vi "Device cluster to publisher cluster.vi"(8 "error in":errorcluster, 9 "Device cluster from subVi/Dll":T3, 11 "old Data cluster":T1) -> (0 "errorout":errorcluster, 3 "Data cluster out":T1)   [LabVIEW 2013]
uses:
  dataCluster.ctl
  <vilib>/vision/Image Controls.llb/IMAQ Image.ctl
  DataQueueTypeDef.ctl
  PolyRead/StringRead.vi
  PolyRead/ErrorRead.vi
  PolyRead/u32Read.vi
  PolyRead/PathRead.vi
  PolyRead/I32Read.vi
  PolyRead/BooleanRead.vi
  PolyRead/I32refRead.vi
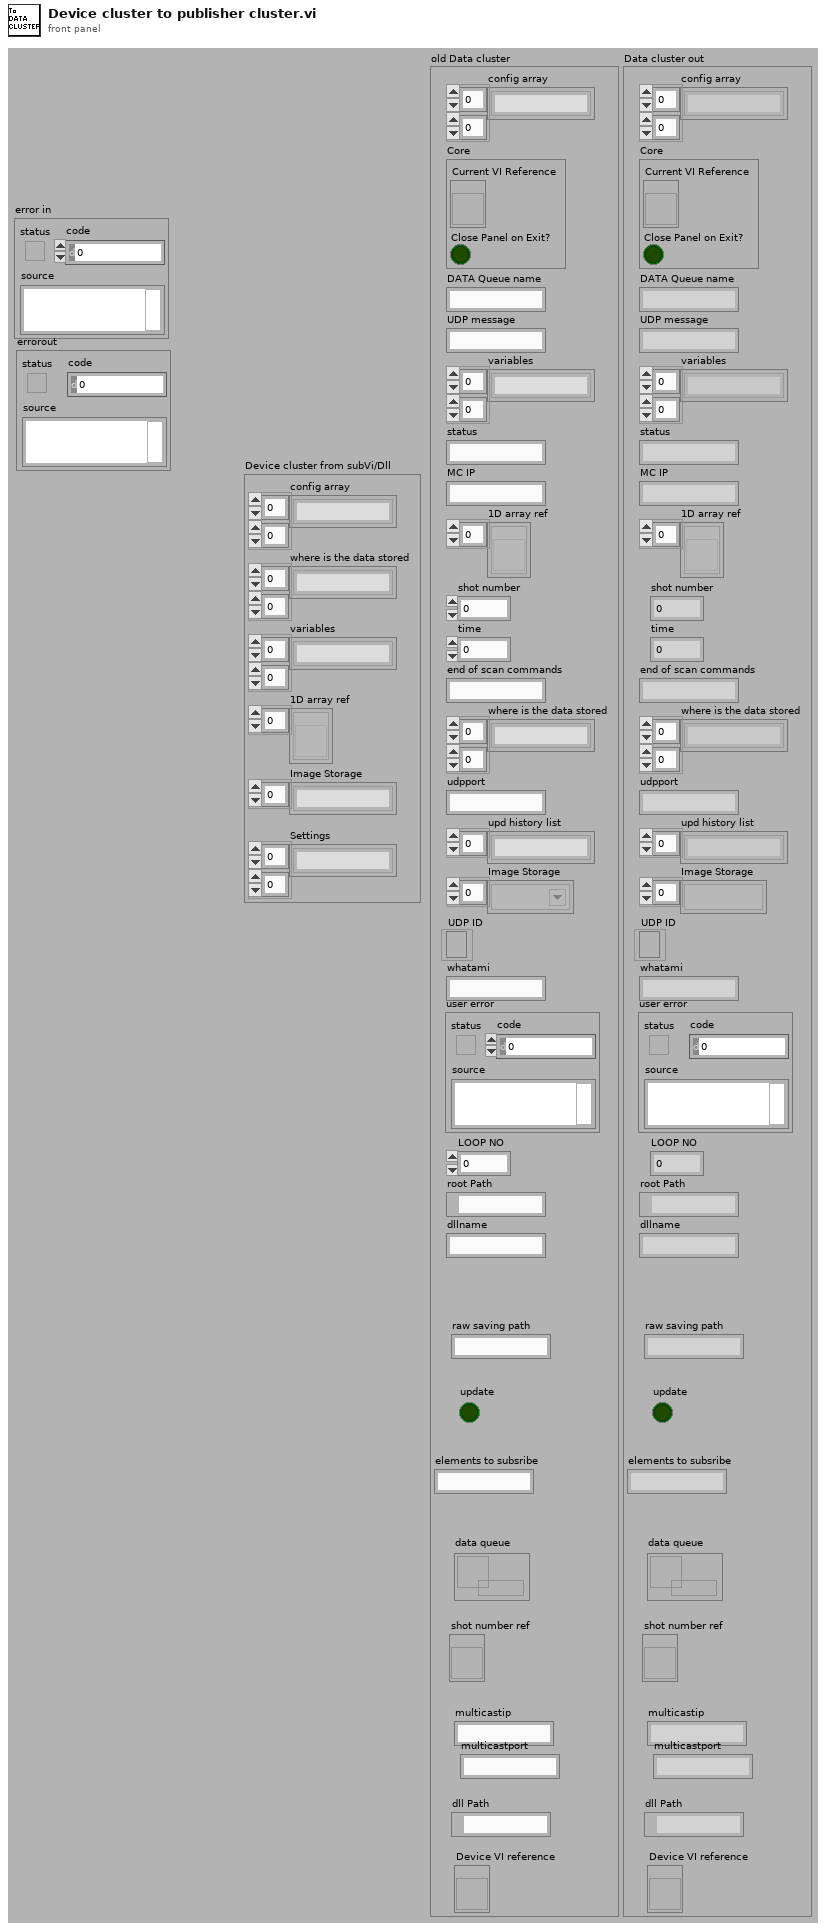
[diagram p1: front panel]
types:
  T1 = typedef "dataCluster.ctl" = cluster{"config array":string[][], "Core":cluster{"Current VI Reference":refnum<vi>, "Close Panel on Exit?":bool}, "DATA Queue name":string, "UDP message":string, "variables":string[][], "status":string, "MC IP":string, "1D array ref":refnum<vi>[], "shot number":i32, "time":u32, "end of scan commands":string, "where is the data stored":string[][], "udpport":string, "upd history list":string[], "Image Storage":T2[], "UDP ID":refnum<k16>, "whatami":string, "user error":errorcluster, "LOOP NO":u32, "root Path":path, "dllname":string, "raw saving path":string, "update":bool, "elements to subsribe":string, "data queue":refnum<queue>, "shot number ref":refnum<vi>, "multicastip":string, "multicastport":string, "dll Path":path, "Device VI reference":refnum<vi>}
  T2 = typedef "IMAQ Image.ctl" = refnum<image>
  T3 = cluster{"config array":string[][], "where is the data stored":string[][], "variables":string[][], "1D array ref":refnum<vi>[], "Image Storage":string[], "Settings":string[][]}
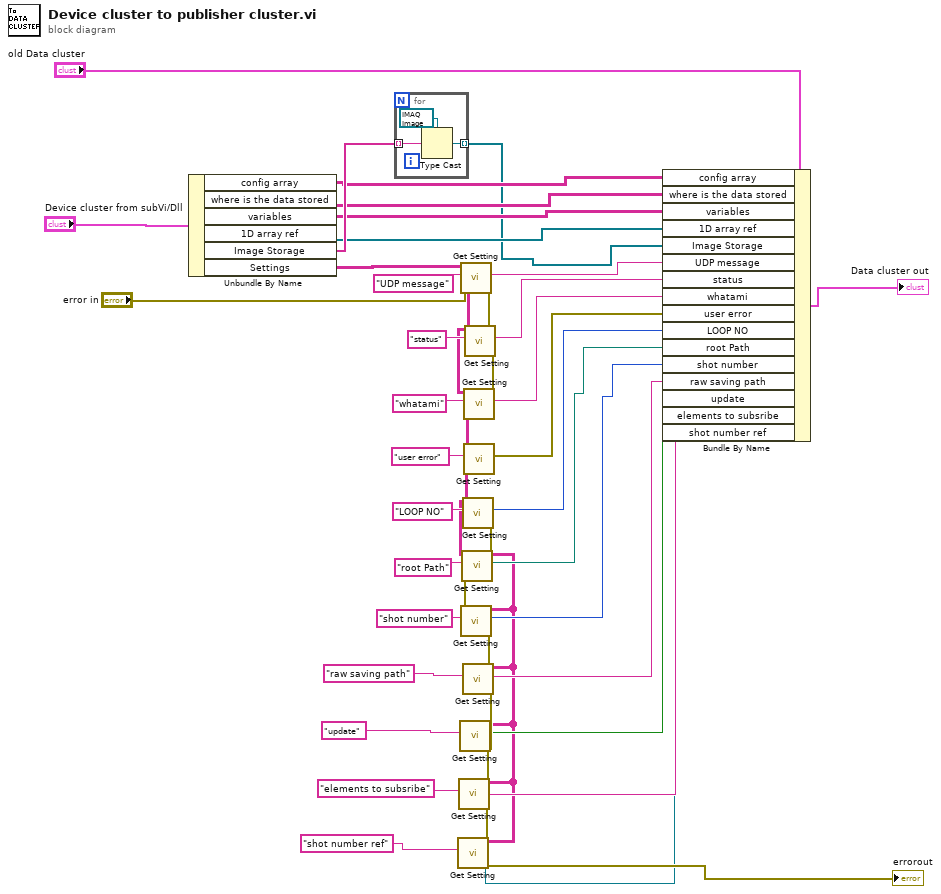
[diagram p0: block diagram]
diagram:
  n1 = Unbundle By Name("Device cluster from subVi/Dll") -> ("config array"=w34:string[][], "where is the data stored"=w33:string[][], "variables"=w32:string[][], "1D array ref"=w31:refnum<vi>[], "Image Storage"=w36:string[], "Settings"=w49:string[][])
  n2 = for {
    tunnel: w36 -> [w53] mode=indexing
    tunnel: [w51] -> w30 mode=indexing
    n3 = Type Cast(type=T2 refnum ("New Image"), x=w53) -> (*(type *) &x=w51:T2)
  }
  n4 = call-poly "Get Setting.vi"("error in"="error in", "Variable Name"="UDP message" ("string"), "array in"=w49) -> ("error out"=w20:errorcluster, "String"=w29:string, "array out"=w41:string[][])  [unwired: 6 in]
  n5 = call-poly "Get Setting.vi"("error in"=w20, "Variable Name"="status" ("string"), "array in"=w41) -> ("error out"=w19:errorcluster, "String"=w28:string, "array out"=w40:string[][])  [unwired: 6 in]
  n6 = call-poly "Get Setting.vi"("error in"=w19, "Variable Name"="whatami", "array in"=w40) -> ("error out"=w18:errorcluster, "String"=w27:string, "array out"=w39:string[][])  [unwired: 6 in]
  n7 = call-poly "Get Setting.vi"("error in"=w18, "Variable Name"="user error", "array in"=w39) -> ("error out"=w17:errorcluster, "error 2"=w26:errorcluster, "array out"=w38:string[][])  [unwired: 6 in]
  n8 = call-poly "Get Setting.vi"("error in"=w17, "Variable Name"="LOOP NO", "array in"=w38) -> ("error out"=w16:errorcluster, "I32 2"=w25:u32, "array out"=w37:string[][])  [unwired: 6 in]
  n9 = call-poly "Get Setting.vi"("error in"=w16, "Variable Name"="root Path", "array in"=w37) -> ("error out"=w15:errorcluster, "Path 2"=w24:path, "array out"=w5:string[][])  [unwired: 6 in]
  n10 = call-poly "Get Setting.vi"("error in"=w15, "Variable Name"="shot number", "array in"=w5) -> ("error out"=w9:errorcluster, "I32 2"=w23:i32)  [unwired: 6 in, 1 out]
  n11 = call-poly "Get Setting.vi"("error in"=w9, "Variable Name"="raw saving path", "array in"=w5) -> ("error out"=w11:errorcluster, "String"=w13:string)  [unwired: 6 in, 1 out]
  n12 = call-poly "Get Setting.vi"("error in"=w11, "Variable Name"="update", "array in"=w5) -> ("error out"=w7:errorcluster, "value"=w10:bool)  [unwired: 6 in, 1 out]
  n13 = call-poly "Get Setting.vi"("error in"=w7, "Variable Name"="elements to subsribe", "array in"=w5) -> ("error out"=w4:errorcluster, "String"=w6:string)  [unwired: 6 in, 1 out]
  n14 = call-poly "Get Setting.vi"("error in"=w4, "Variable Name"="shot number ref", "array in"=w5) -> ("error out"=→"errorout":errorcluster, "I32ref"=w1:refnum<vi>)  [unwired: 6 in, 1 out]
  n15 = Bundle By Name(cluster="old Data cluster", "config array"=w34, "where is the data stored"=w33, "variables"=w32, "1D array ref"=w31, "Image Storage"=w30, "UDP message"=w29, "status"=w28, "whatami"=w27, "user error"=w26, "LOOP NO"=w25, "root Path"=w24, "shot number"=w23, "raw saving path"=w13, "update"=w10, "elements to subsribe"=w6, "shot number ref"=w1) -> (→"Data cluster out":T1)
